vi "20220114 vision item position.vi"(8 "error in":errorcluster) -> (0 "error out":errorcluster, 3 "Numeric":dbl)   [LabVIEW 2019]
panel:
  out "Image Out":T1(plugin-control)
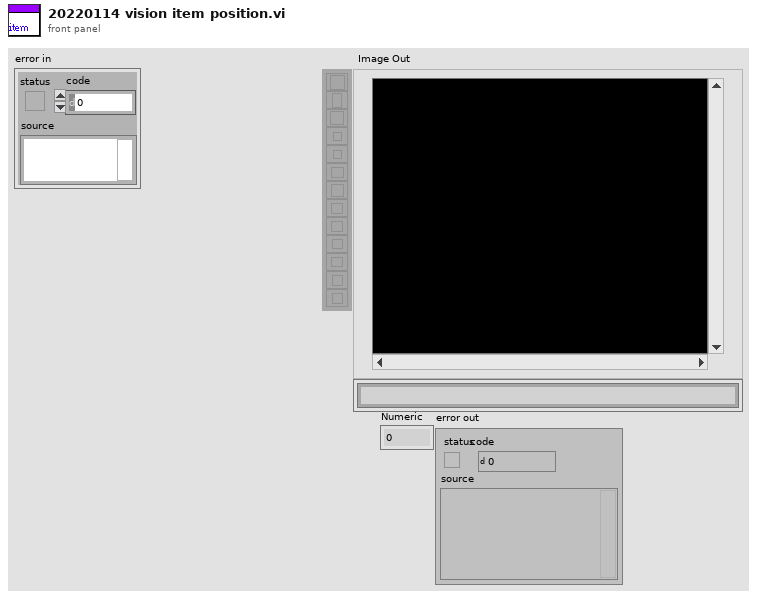
[diagram p1: front panel]
types:
  T1 = typedef "IMAQ Image.ctl" = refnum<image>
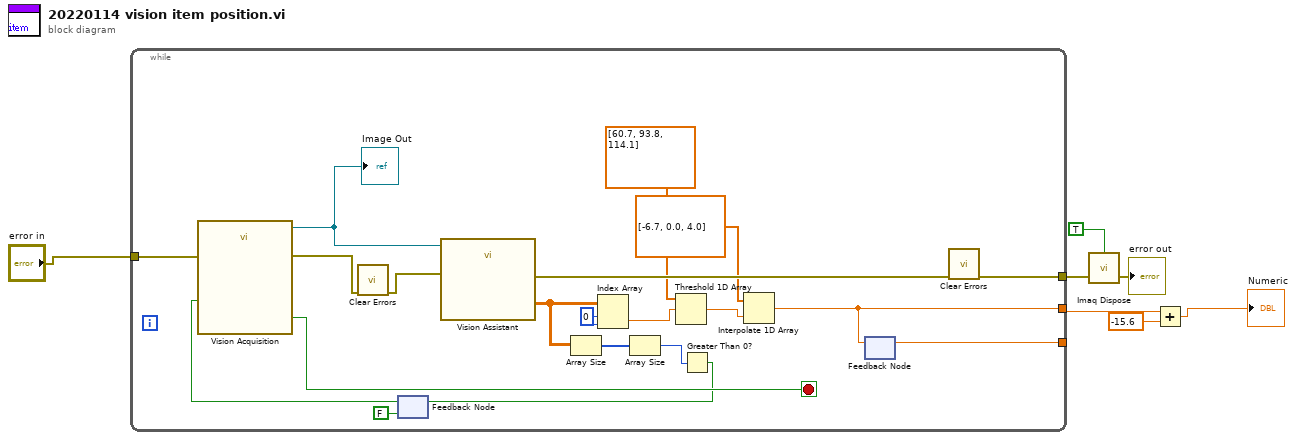
[diagram p0: block diagram]
diagram:
  n1 = while {
    tunnel: [w8] -> w7
    tunnel: [w13] -> w5
    tunnel: [w12] -> _
    tunnel: "error in" -> [w11]
    stop <- w27 stop-if-true
    w24 = 0 ("index (row)")
    n2 = feedback #1(FALSE) -> (w15:bool)
    n3 = call "Vision Acquisition"("Stop (F)"=w15, "error in"=w11) -> ("Image Out"=w26:T1, "Stopped"=w27:bool, "error out"=w10:errorcluster)  [unwired: 23 in]
    "Image Out" <- w26
    n4 = call <vilib>:"Clear Errors.vi"("error in (no error)"=w10) -> ("error out"=w9:errorcluster)  [unwired: 5 in, 1 out]
    n5 = call "Vision Assistant"("Image In"=w26, "error in"=w9) -> ("Particle Measurements (Pixels) (Particle Analysis 1)"=w19:dbl[][], "error out"=w25:errorcluster)  [unwired: 23 in, 1 out]
    n6 = Array Size(array=w19) -> (size(s)=w18:i32[])
    n7 = Index Array(array=w19, index (row)=w24, index (col)=w24) -> (element=w23:dbl)
    n8 = Array Size(array=w18) -> (size(s)=w17:i32)
    n9 = Threshold 1D Array(2:w23, 3:dbl[] [60.7, 93.8, 114.1]) -> (0:w20:dbl)  [unwired: 1 in]
    n10 = Greater Than 0?(x=w17) -> (x > 0?=w16:bool)
    n11 = feedback-in #1(w16) -> ()
    n12 = Interpolate 1D Array(1:w20, 2:dbl[] [-6.7, 0.0, 4.0]) -> (0:w13:dbl)
    n13 = feedback-in #2(w13) -> ()
    n14 = feedback #2() -> (w12:dbl)  [unwired: 1 in]
    n15 = call <vilib>:"Clear Errors.vi"("error in (no error)"=w25) -> ("error out"=w8:errorcluster)  [unwired: 5 in, 1 out]
  }
  n16 = call "Imaq Dispose"("All Images? (No)"=TRUE, "error in (no error)"=w7) -> ("error out"=→"error out":errorcluster)  [unwired: 4 in]
  n17 = Add(x=w5, y=-15.6) -> (x+y=→"Numeric":dbl)
